vi "Configuration.vi"() -> ()   [LabVIEW 2019]
uses:
  Sub VIs/Configuration/Configuration.ctl
panel:
  in  "Stop Program":bool
  in  "Save Configuration":bool
  in  "Load Saved Configuration":bool
  in  "Configuration":T1={"Accelerometer Bias"={"X (m/s)"=0.0, "Y (m/s)"=0.0, "Z (m/s)"=0.0}, "Gyroscope Bias"={"X (m/s)"=0.0, "Y (m/s)"=0.0, "Z (m/s)"=0.0}, "Steering Motor Gear Ratio"=611.0, "Steering Pully Gear Ratio"=1.0, "Steering Encoder CPR"=500.0, "Steering Motor Max RPM"=4000.0, "Wheelbase (m)"=1.12, "Fork Angle (rad)"=1.3, "Balancing Controller"={"Kp (/s)"=0.5, "Kd (1)"=0.0}, "Max Allowed Steering Angle (rad)"=0.7, "Task Periods"={"Emergency Stop (us)"=10000, "IMU (us)"=10000, "Steering Motor Encoder (us)"=10000, "State Estimator (us)"=10000, "Balancing Controller (us)"=10000, "GNSS (us)"=10000, "Logging (us)"=10000}}
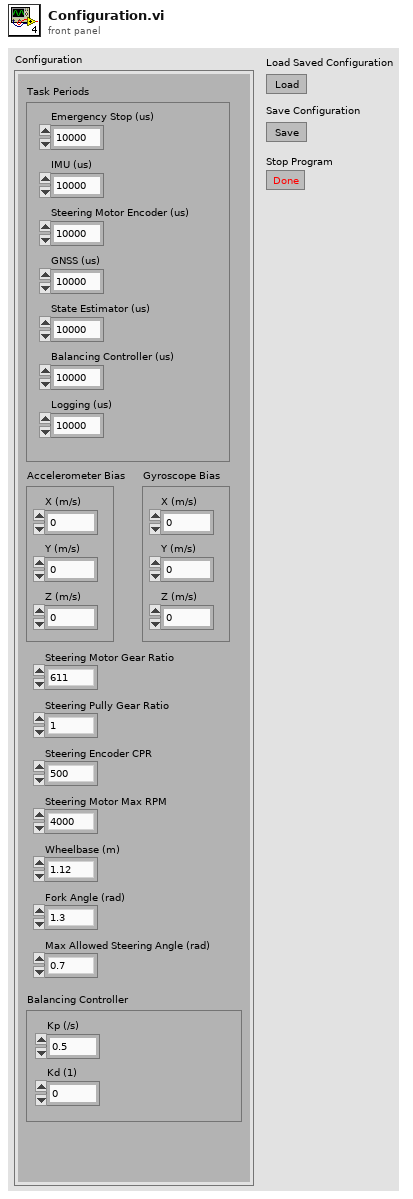
[diagram p1: front panel]
types:
  T1 = typedef "Configuration.ctl" = cluster{"Accelerometer Bias":cluster{"X (m/s)":dbl, "Y (m/s)":dbl, "Z (m/s)":dbl}, "Gyroscope Bias":cluster{"X (m/s)":dbl, "Y (m/s)":dbl, "Z (m/s)":dbl}, "Steering Motor Gear Ratio":dbl, "Steering Pully Gear Ratio":dbl, "Steering Encoder CPR":dbl, "Steering Motor Max RPM":dbl, "Wheelbase (m)":dbl, "Fork Angle (rad)":dbl, "Balancing Controller":cluster{"Kp (/s)":dbl, "Kd (1)":dbl}, "Max Allowed Steering Angle (rad)":dbl, "Task Periods":cluster{"Emergency Stop (us)":i64, "IMU (us)":i64, "Steering Motor Encoder (us)":i64, "State Estimator (us)":i64, "Balancing Controller (us)":i64, "GNSS (us)":i64, "Logging (us)":i64}}
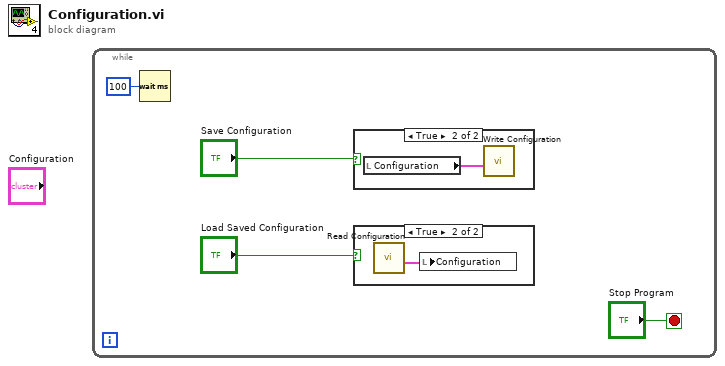
[diagram p0: block diagram]
diagram:
  n1 = while {
    stop <- "Stop Program" stop-if-true
    n2 = Wait (ms)(milliseconds to wait=u32 100) -> ()  [unwired: 1 out]
    n3 = case shown="True" "Save Configuration" {
      frame False {
      }
      frame True {
        n4 = local read "Configuration"() -> (w5:T1)
        n5 = call "Write Configuration.vi"("Configuration"=w5) -> ()  [unwired: 10 in, 1 out]
      }
    }
    n6 = case shown="True" "Load Saved Configuration" {
      frame False {
      }
      frame True {
        n7 = call "Read Configuration.vi"() -> ("Configuration"=w6:T1)  [unwired: 10 in, 1 out]
        n8 = local write "Configuration"(w6) -> ()
      }
    }
  }
